vi "AC Build Graph.vi"(9 "Inputs":T1, 10 "Numeric":dbl, 11 "Array in":dbl[][](array[numeric])) -> (3 "Array out":dbl[][](array[numeric]))   [LabVIEW 2017]
uses:
  controls/All Inputs.ctl
  controls/SACB DI.ctl
panel:
  in  "Average?":bool
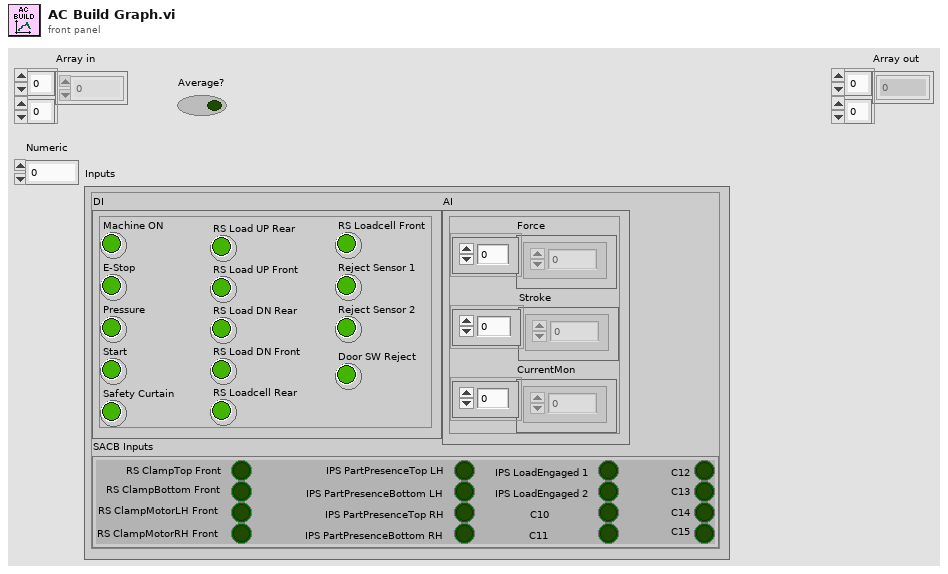
[diagram p1: front panel]
types:
  T1 = typedef "All Inputs.ctl" = cluster{"DI":cluster{"Machine ON":bool, "E-Stop":bool, "Pressure":bool, "Start":bool, "Safety Curtain":bool, "RS Load UP Rear":bool, "RS Load UP Front":bool, "RS Load DN Rear":bool, "RS Load DN Front":bool, "RS Loadcell Rear":bool, "RS Loadcell Front":bool, "Reject Sensor 1":bool, "Reject Sensor 2":bool, "Door SW Reject":bool}, "AI":cluster{"Force":dbl[], "Stroke":dbl[], "CurrentMon":dbl[]}, "SACB Inputs":T2}
  T2 = typedef "SACB DI.ctl" = cluster{"RS ClampTop Front":bool, "RS ClampBottom Front":bool, "RS ClampMotorLH Front":bool, "RS ClampMotorRH Front":bool, "IPS PartPresenceTop LH":bool, "IPS PartPresenceBottom LH":bool, "IPS PartPresenceTop RH":bool, "IPS PartPresenceBottom RH":bool, "IPS LoadEngaged 1":bool, "IPS LoadEngaged 2":bool, "C10":bool, "C11":bool, "C12":bool, "C13":bool, "C14":bool, "C15":bool}
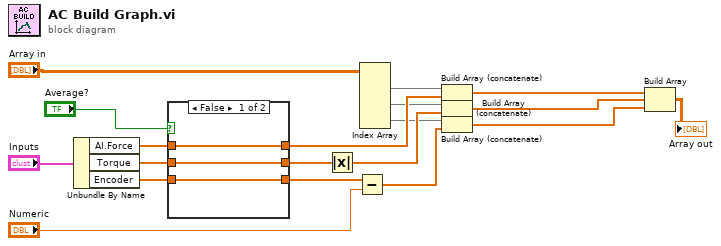
[diagram p0: block diagram]
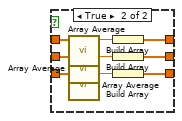
[diagram p2: hidden frame]
diagram:
  n1 = Unbundle By Name("Inputs") -> ("AI.Force"=w12:dbl[], "Torque"=w14:dbl[], "Encoder"=w15:dbl[])
  n2 = case shown="False" "Average?" {
    tunnel: [w21 w24] -> w17
    tunnel: [w22 w23] -> w16
    tunnel: w15 -> [w22 w29]
    tunnel: w14 -> [w21 w28]
    tunnel: [w20 w25] -> w13
    tunnel: w12 -> [w20 w26]
    frame False {
    }
    frame True {
      n3 = call "Array Average.vi"("data"=w26) -> ("Numeric"=w27:dbl)  [unwired: 10 in]
      n4 = call "Array Average.vi"("data"=w28) -> ("Numeric"=w31:dbl)  [unwired: 10 in]
      n5 = call "Array Average.vi"("data"=w29) -> ("Numeric"=w30:dbl)  [unwired: 10 in]
      n6 = Build Array(w27) -> (w25:dbl[])
      n7 = Build Array(w31) -> (w24:dbl[])
      n8 = Build Array(w30) -> (w23:dbl[])
    }
  }
  n9 = Absolute Value(x=w17) -> (abs(x)=w9:dbl[])
  n10 = Subtract(x=w16, y="Numeric") -> (x-y=w11:dbl[])
  n11 = Index Array(array="Array in") -> (element #1=w3:dbl[], element #2=w4:dbl[], element #3=w5:dbl[])  [unwired: 6 in]
  n12 = Build Array (concatenate)(w3, w13) -> (w6:dbl[])
  n13 = Build Array (concatenate)(w4, w9) -> (w18:dbl[])
  n14 = Build Array (concatenate)(w5, w11) -> (w7:dbl[])
  n15 = Build Array(w6, w18, w7) -> (→"Array out":dbl[][])
